vi "IB_RW_Project_Clear_Source.vi"(8 "error in (no error)":errorcluster, 11 "buildObject":T1) -> (0 "error out":errorcluster, 3 "buildObject out":T1)   [LabVIEW 2020]
doc: "Reads and writes the data to the object property bag."
uses:
  <vilib>/AppBuilder/IB_RW_Project/IB_RW_Project_PropBag_Action.ctl
  <resource>/Framework/Providers/API/ItemRef.ctl
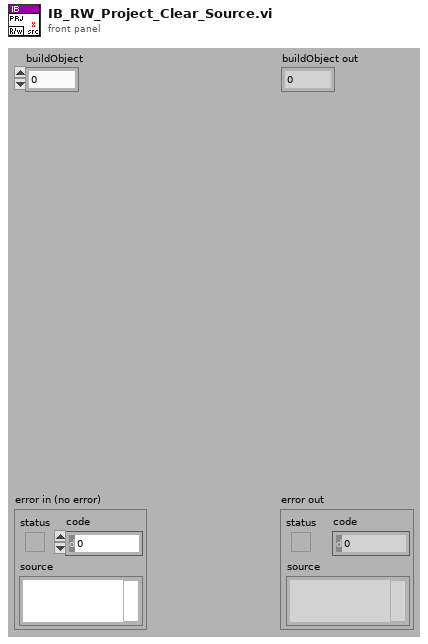
[diagram p1: front panel]
types:
  T1 = typedef "ItemRef.ctl" = u64
  T2 = typedef "IB_RW_Project_PropBag_Action.ctl" = enum16{"read", "write", "clear", "readPrevious", "writePrevious", "clearPrevious"}
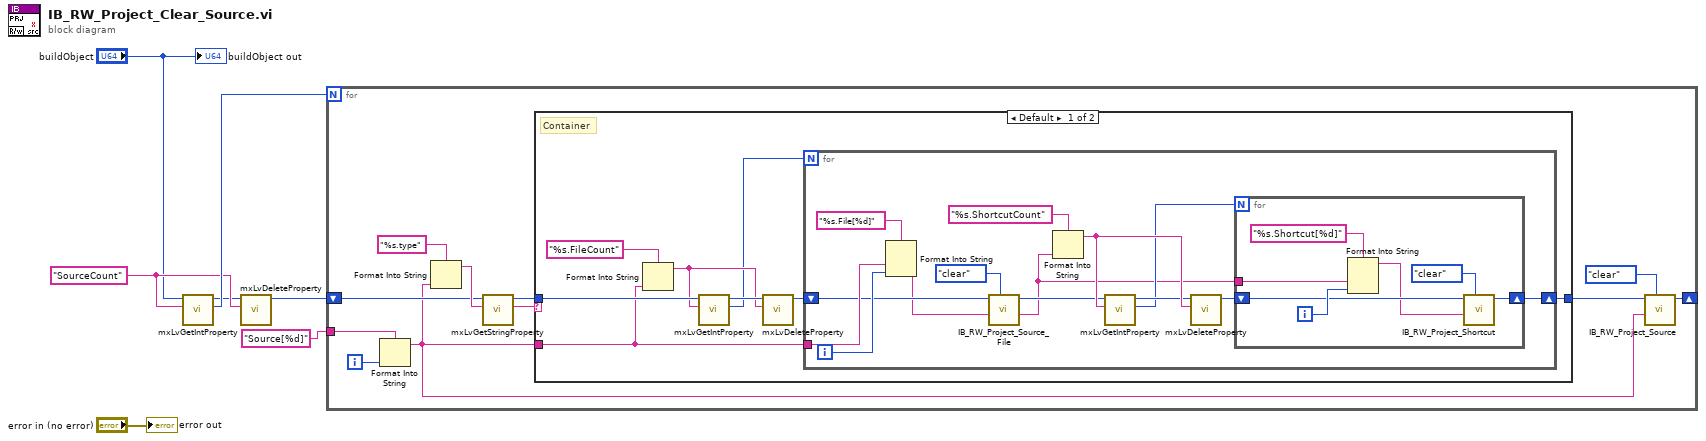
[diagram p0: block diagram]
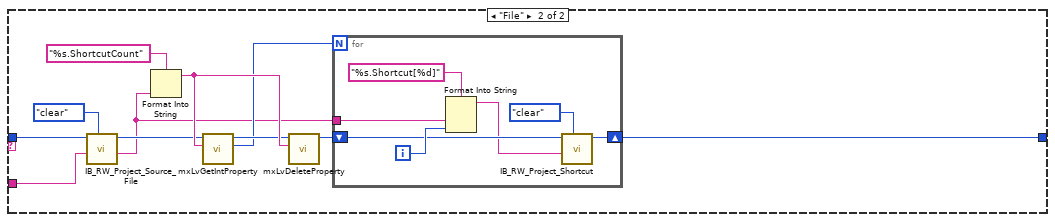
[diagram p2: hidden frame]
diagram:
  w6 = "SourceCount"
  n1 = call <resource>:"mxLvGetIntProperty.vi"("Tag"=w6, "Item"="buildObject") -> ("Value"=w7:i32, "Item"=w5:T1)  [unwired: 1 in, 7 out]
  n2 = call <resource>:"mxLvDeleteProperty.vi"("Tag"=w6, "Item"=w5) -> ("Item"=w4:T1)  [unwired: 1 in, 8 out]
  n3 = for {
    N: w7 -> [_]
    shift-right: [w10] -> _
    shift-left: w4 -> [w9]
    tunnel: "Source[%d]" -> [w17]
    i -> [w18]
    n4 = Format Into String(format string=w17, w18) -> (resulting string=w8:string)  [unwired: 2 in, 1 out]
    n5 = Format Into String(format string="%s.type", w8) -> (resulting string=w14:string)  [unwired: 2 in, 1 out]
    n6 = call <resource>:"mxLvGetStringProperty.vi"("Tag"=w14, "Item"=w9) -> ("Value"=w15:string, "Item"=w13:T1)  [unwired: 1 in, 7 out]
    n7 = case shown="Default" w15 {
      tunnel: w13 -> [w25 w57]
      tunnel: [w20 w50] -> w11
      tunnel: w8 -> [w19 w56]
      frame Default {
        # "Container"
        n8 = Format Into String(format string="%s.FileCount", w19) -> (resulting string=w23:string)  [unwired: 2 in, 1 out]
        n9 = call <resource>:"mxLvGetIntProperty.vi"("Tag"=w23, "Item"=w25) -> ("Value"=w22:i32, "Item"=w24:T1)  [unwired: 1 in, 7 out]
        n10 = call <resource>:"mxLvDeleteProperty.vi"("Tag"=w23, "Item"=w24) -> ("Item"=w21:T1)  [unwired: 1 in, 8 out]
        n11 = for {
          N: w22 -> [_]
          shift-right: [w27] -> w20
          shift-left: w21 -> [w29]
          tunnel: w19 -> [w38]
          i -> [w39]
          n12 = Format Into String(format string="%s.File[%d]", w38, w39) -> (resulting string=w28:string)  [unwired: 2 in, 1 out]
          n13 = call <vilib>:"IB_RW_Project_Source_File.vi"("action"=IB_RW_Project_PropBag_Action."clear", "index in"=w28, "buildObject"=w29) -> ("index out"=w30:string, "buildObject out"=w33:T1)  [unwired: 5 in, 2 out]
          n14 = Format Into String(format string="%s.ShortcutCount", w30) -> (resulting string=w35:string)  [unwired: 2 in, 1 out]
          n15 = call <resource>:"mxLvGetIntProperty.vi"("Tag"=w35, "Item"=w33) -> ("Value"=w31:i32, "Item"=w34:T1)  [unwired: 1 in, 7 out]
          n16 = call <resource>:"mxLvDeleteProperty.vi"("Tag"=w35, "Item"=w34) -> ("Item"=w32:T1)  [unwired: 1 in, 8 out]
          n17 = for {
            N: w31 -> [_]
            shift-right: [w42] -> w27
            shift-left: w32 -> [w43]
            tunnel: w30 -> [w46]
            i -> [w45]
            n18 = Format Into String(format string="%s.Shortcut[%d]", w46, w45) -> (resulting string=w41:string)  [unwired: 2 in, 1 out]
            n19 = call <vilib>:"IB_RW_Project_Shortcut.vi"("action"=IB_RW_Project_PropBag_Action."clear", "index in"=w41, "buildObject"=w43) -> ("buildObject out"=w42:T1)  [unwired: 5 in, 3 out]
          }
        }
      }
      frame "File" {
        n20 = call <vilib>:"IB_RW_Project_Source_File.vi"("action"=IB_RW_Project_PropBag_Action."clear", "index in"=w56, "buildObject"=w57) -> ("index out"=w48:string, "buildObject out"=w52:T1)  [unwired: 5 in, 2 out]
        n21 = Format Into String(format string="%s.ShortcutCount", w48) -> (resulting string=w54:string)  [unwired: 2 in, 1 out]
        n22 = call <resource>:"mxLvGetIntProperty.vi"("Tag"=w54, "Item"=w52) -> ("Value"=w49:i32, "Item"=w53:T1)  [unwired: 1 in, 7 out]
        n23 = call <resource>:"mxLvDeleteProperty.vi"("Tag"=w54, "Item"=w53) -> ("Item"=w51:T1)  [unwired: 1 in, 8 out]
        n24 = for {
          N: w49 -> [_]
          shift-right: [w60] -> w50
          shift-left: w51 -> [w61]
          tunnel: w48 -> [w64]
          i -> [w63]
          n25 = Format Into String(format string="%s.Shortcut[%d]", w64, w63) -> (resulting string=w59:string)  [unwired: 2 in, 1 out]
          n26 = call <vilib>:"IB_RW_Project_Shortcut.vi"("action"=IB_RW_Project_PropBag_Action."clear", "index in"=w59, "buildObject"=w61) -> ("buildObject out"=w60:T1)  [unwired: 5 in, 3 out]
        }
      }
    }
    n27 = call <vilib>:"IB_RW_Project_Source.vi"("action"=IB_RW_Project_PropBag_Action."clear", "index in"=w8, "buildObject"=w11) -> ("buildObject out"=w10:T1)  [unwired: 5 in, 3 out]
  }
  "error out" <- "error in (no error)"
  "buildObject out" <- "buildObject"
